vi "WriteConfiguration_FP.vi"(8 "error in":errorcluster, 11 "PythonConverter_GUI in":refnum<class "PythonConverter_GUI.lvclass">) -> (0 "error out":errorcluster, 3 "PythonConverter_GUI out":refnum<class "PythonConverter_GUI.lvclass">)   [LabVIEW 2014, in "PythonConverter_GUI.lvclass"]
uses:
  PythonConverter_GUI.lvclass
  PythonConverter_GUI.lvclass/PythonConverter_GUI.ctl
  VI Interpreter/Classes/VI Interpreter/VI Interpreter.lvclass/VI Interpreter.ctl
  PythonConfiguration/PythonConfiguration.lvclass/PythonConfiguration.ctl
  VI Interpreter/Classes/FPWindow/FPWindow.lvclass/FPWindow.ctl
  <vilib>/Utility/miscctls.llb/LVPointTypeDef.ctl
  VI Interpreter/Classes/VI Interpreter/VI Interpreter.lvclass
  VI Interpreter/Classes/FPWindow/FPWindow.lvclass
  PythonConfiguration/PythonConfiguration.lvclass
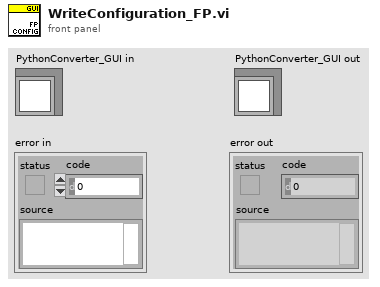
[diagram p1: front panel]
types:
  T1 = typedef "LVPointTypeDef.ctl" = cluster{"Horizontal":i16, "Vertical":i16}
  T2 = typedef "PythonConfiguration.lvclass/ItemTD.ctl" = cluster{"Key":string, "Value":string}
  T3 = typedef "LVRectTypeDef.ctl" = cluster{"Left":i16, "Top":i16, "Right":i16, "Bottom":i16}
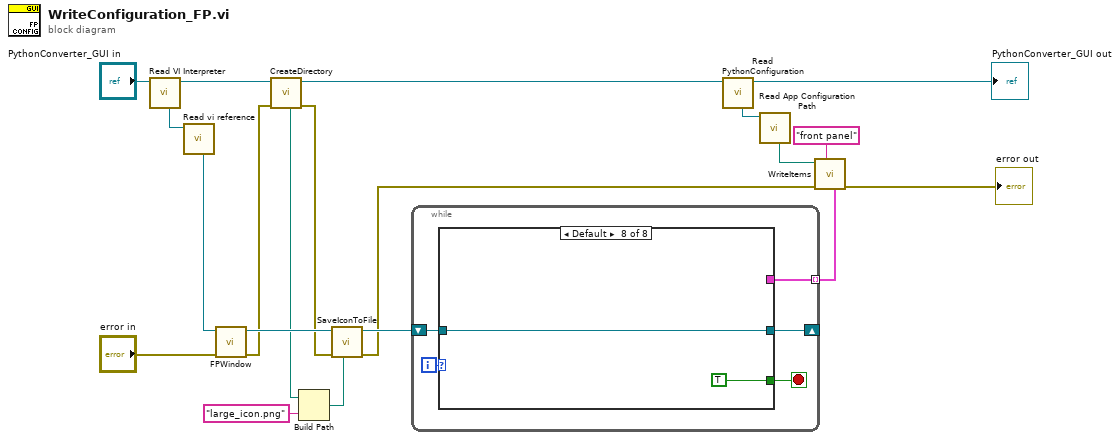
[diagram p0: block diagram]
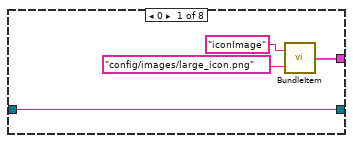
[diagram p2: hidden frame]
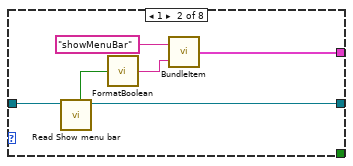
[diagram p3: hidden frame]
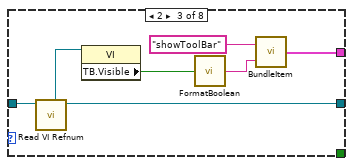
[diagram p4: hidden frame]
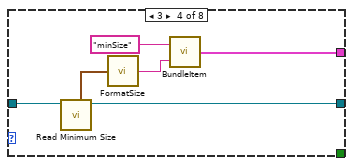
[diagram p5: hidden frame]
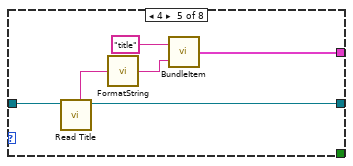
[diagram p6: hidden frame]
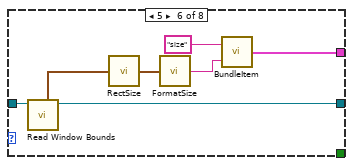
[diagram p7: hidden frame]
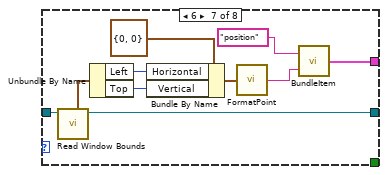
[diagram p8: hidden frame]
diagram:
  n1 = call "Read VI Interpreter.vi"("PythonConverter_GUI in"="PythonConverter_GUI in") -> ("PythonConverter_GUI out"=w2:refnum<class "PythonConverter_GUI.lvclass">, "VI Interpreter"=w1:refnum<class "VI Interpreter.lvclass">)  [unwired: 7 in]
  n2 = call "Read vi reference.vi"("VI Interpreter in"=w1) -> ("vi reference"=w19:refnum<vi>)  [unwired: 7 in, 1 out]
  n3 = call "FPWindow.vi"("error in"="error in", "VI Refnum"=w19) -> ("error out"=w17:errorcluster, "FPWindow out"=w18:refnum<class "FPWindow.lvclass">)  [unwired: 8 in]
  n4 = call "CreateDirectory.vi"("error in"=w17, "PythonConverter_GUI in"=w2) -> ("error out"=w16:errorcluster, "PythonConverter_GUI out"=w13:refnum<class "PythonConverter_GUI.lvclass">, "Path"=w5:path)  [unwired: 5 in]
  n5 = Build Path(base path=w5, name or relative path="large_icon.png") -> (appended path=w4:path)
  n6 = call "SaveIconToFile.vi"("Image File"=w4, "error in"=w16, "FPWindow in"=w18) -> ("error out"=w8:errorcluster, "FPWindow out"=w12:refnum<class "FPWindow.lvclass">)  [unwired: 5 in]
  n7 = while {
    shift-right: [w23] -> _
    shift-left: w12 -> [w24]
    tunnel: [w22] -> w11 mode=indexing
    i -> [w25]
    stop <- w21 stop-if-true
    n8 = case shown="Default" w25 {
      tunnel: w24 -> [w26 w32 w40 w45 w52 w59 w69 w73]
      tunnel: [w26 w31 w39 w44 w51 w58 w68 w73] -> w23
      tunnel: [w28 w30 w38 w43 w50 w57 w67 _] -> w22
      tunnel: [_ _ _ _ _ _ _ TRUE] -> w21
      frame 0 {
        n9 = call "BundleItem.vi"("Value"="config/images/large_icon.png", "Key"="iconImage") -> ("Item"=w28:T2)
      }
      frame 1 {
        n10 = call "Read Show menu bar.vi"("FPWindow in"=w32) -> ("FPWindow out"=w31:refnum<class "FPWindow.lvclass">, "Show menu bar"=w33:bool)  [unwired: 7 in]
        n11 = call "FormatBoolean.vi"("boolean"=w33) -> ("value"=w34:string)
        n12 = call "BundleItem.vi"("Value"=w34, "Key"="showMenuBar") -> ("Item"=w30:T2)
      }
      frame 2 {
        n13 = call "Read VI Refnum.vi"("FPWindow in"=w40) -> ("FPWindow out"=w39:refnum<class "FPWindow.lvclass">, "VI Refnum"=w36:refnum<vi>)  [unwired: 7 in]
        n14 = property class="VI"(reference=w36) -> ("TB.Visible"=w37:bool)  [unwired: 1 in, 2 out]
        n15 = call "FormatBoolean.vi"("boolean"=w37) -> ("value"=w41:string)
        n16 = call "BundleItem.vi"("Value"=w41, "Key"="showToolBar") -> ("Item"=w38:T2)
      }
      frame 3 {
        n17 = call "Read Minimum Size.vi"("FPWindow in"=w45) -> ("FPWindow out"=w44:refnum<class "FPWindow.lvclass">, "Minimum Size"=w46:T1)  [unwired: 7 in]
        n18 = call "FormatSize.vi"("size"=w46) -> ("value"=w47:string)
        n19 = call "BundleItem.vi"("Value"=w47, "Key"="minSize") -> ("Item"=w43:T2)
      }
      frame 4 {
        n20 = call "Read Title.vi"("FPWindow in"=w52) -> ("FPWindow out"=w51:refnum<class "FPWindow.lvclass">, "Title"=w49:string)  [unwired: 7 in]
        n21 = call "FormatString.vi"("String"=w49) -> ("value"=w53:string)  [unwired: 1 in]
        n22 = call "BundleItem.vi"("Value"=w53, "Key"="title") -> ("Item"=w50:T2)
      }
      frame 5 {
        n23 = call "Read Window Bounds.vi"("FPWindow in"=w59) -> ("FPWindow out"=w58:refnum<class "FPWindow.lvclass">, "Panel Bounds"=w55:T3)  [unwired: 7 in]
        n24 = call <vilib>:"RectSize.vi"("rect"=w55) -> ("point"=w56:cluster{"x":i16, "y":i16})
        n25 = call "FormatSize.vi"("size"=w56) -> ("value"=w60:string)
        n26 = call "BundleItem.vi"("Value"=w60, "Key"="size") -> ("Item"=w57:T2)
      }
      frame 6 {
        n27 = call "Read Window Bounds.vi"("FPWindow in"=w69) -> ("FPWindow out"=w68:refnum<class "FPWindow.lvclass">, "Panel Bounds"=w64:T3)  [unwired: 7 in]
        n28 = Unbundle By Name(w64) -> ("Left"=w63:i16, "Top"=w62:i16)
        n29 = Bundle By Name(cluster=T1 {"Horizontal"=0, "Vertical"=0} ("point"), "Horizontal"=w63, "Vertical"=w62) -> (w65:T1)
        n30 = call "FormatPoint.vi"("point"=w65) -> ("value"=w70:string)
        n31 = call "BundleItem.vi"("Value"=w70, "Key"="position") -> ("Item"=w67:T2)
      }
      frame Default {
      }
    }
  }
  n32 = call "Read PythonConfiguration.vi"("PythonConverter_GUI in"=w13) -> ("PythonConverter_GUI out"=→"PythonConverter_GUI out":refnum<class "PythonConverter_GUI.lvclass">, "PythonConfiguration"=w14:refnum<class "PythonConfiguration.lvclass">)  [unwired: 7 in]
  n33 = call "Read App Configuration Path.vi"("PythonConfiguration in"=w14) -> ("App Configuration Path"=w15:path)  [unwired: 7 in, 1 out]
  n34 = call "WriteItems.vi"("Items"=w11, "section"="front panel", "error in"=w8, "Path"=w15) -> ("error out"=→"error out":errorcluster)  [unwired: 5 in]
